vi "Shutdown.vi"(8 "error in (no error)":errorcluster, 11 "Framework in":refnum<class "Framework.lvclass">) -> (0 "error out":errorcluster, 3 "Framework out":refnum<class "Framework.lvclass">)   [LabVIEW 2019, in "DSF Core.lvlib" / "Framework.lvclass"]
uses:
  Framework.lvclass
  Framework States.ctl
  Framework.lvclass/Framework.ctl
  Thread Manager/Thread Manager.lvclass
  Interface/Dispatcher/Dispatcher Interface.lvclass
  Interface/Logging/Logging Interface.lvclass
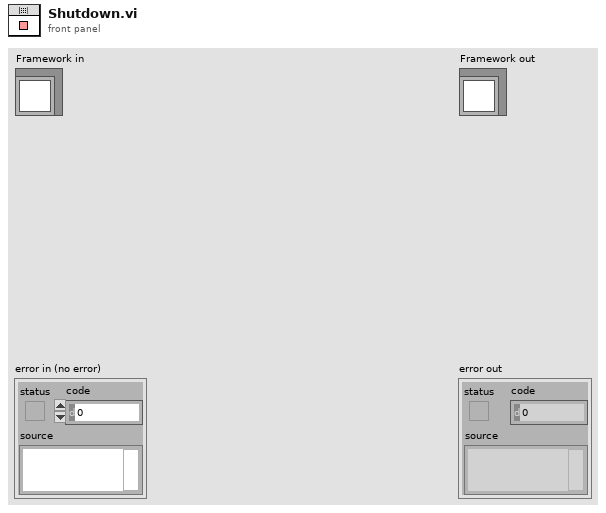
[diagram p1: front panel]
types:
  T1 = typedef "DSF Core.lvlib/Framework.lvclass/Framework States.ctl" = enum8{"Uninitialized", "Initialized", "Start", "Rx", "Tx", "Shutdown"}
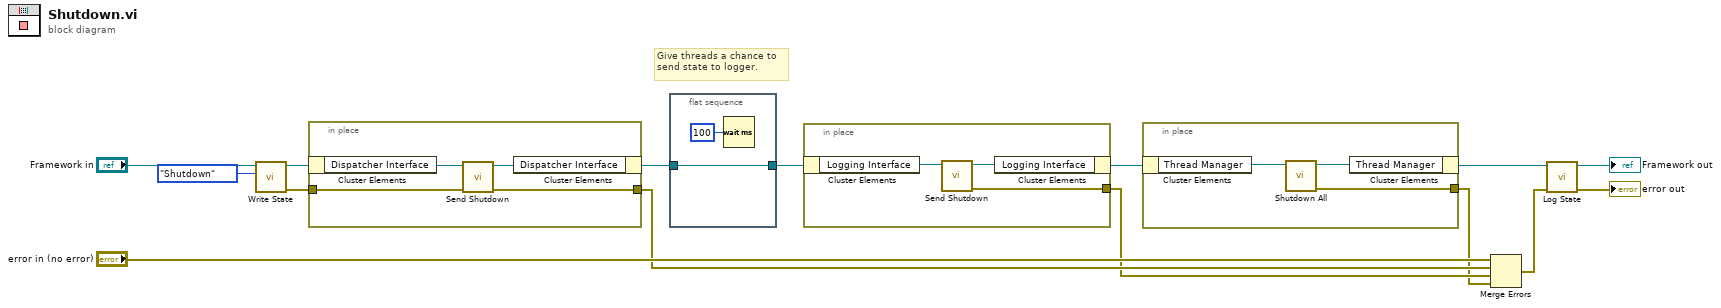
[diagram p0: block diagram]
diagram:
  # "Give threads a chance to send state to logger."
  n1 = call "Write State.vi"("state"=Framework_States."Shutdown", "Framework in"="Framework in") -> ("error out"=w5:errorcluster, "Framework out"=w6:refnum<class "Framework.lvclass">)  [unwired: 8 in]
  n2 = in-place {
    in-place-border: [w17] -> w11
    in-place-border: w5 -> [w16]
    n3 = in-place-cluster #1(w6) -> ("Dispatcher Interface"=w19:refnum<class "Dispatcher Interface.lvclass">)
    n4 = call "Send Shutdown.vi"("error in (no error)"=w16, "Dispatcher Interface in"=w19) -> ("error out"=w17:errorcluster, "Dispatcher Interface out"=w18:refnum<class "Dispatcher Interface.lvclass">)  [unwired: 8 in]
    n5 = in-place-cluster #1("Dispatcher Interface"=w18) -> (w14:refnum<class "Framework.lvclass">)
  }
  n6 = flat-sequence {
    tunnel: w14 -> [w21]
    tunnel: [w21] -> w15
    frame #0 {
      n7 = Wait (ms)(milliseconds to wait=u32 100) -> ()  [unwired: 1 out]
    }
  }
  n8 = in-place {
    in-place-border: [w23] -> w10
    n9 = in-place-cluster #2(w15) -> ("Logging Interface"=w22:refnum<class "Logging Interface.lvclass">)
    n10 = call "Send Shutdown.vi"("Logging Interface in"=w22) -> ("error out"=w23:errorcluster, "Logging Interface out"=w24:refnum<class "Logging Interface.lvclass">)  [unwired: 9 in]
    n11 = in-place-cluster #2("Logging Interface"=w24) -> (w13:refnum<class "Framework.lvclass">)
  }
  n12 = in-place {
    in-place-border: [w25] -> w9
    n13 = in-place-cluster #3(w13) -> ("Thread Manager"=w27:refnum<class "Thread Manager.lvclass">)
    n14 = call "Shutdown All.vi"("Thread Manager in"=w27) -> ("error out"=w25:errorcluster, "Thread Manager out"=w26:refnum<class "Thread Manager.lvclass">)  [unwired: 9 in]
    n15 = in-place-cluster #3("Thread Manager"=w26) -> (w4:refnum<class "Framework.lvclass">)
  }
  n16 = Merge Errors("error in (no error)", w11, w10, w9) -> (w3:errorcluster)
  n17 = call "Log State.vi"("error in (no error)"=w3, "Framework in"=w4) -> ("error out"=→"error out":errorcluster, "Framework out"=→"Framework out":refnum<class "Framework.lvclass">)  [unwired: 8 in]
